vi "Fetch&Process_Measurements_V4.vi"(0 "DCPowerInformation_byChannel":T1(array[cluster]), 5 "Initial Time":timestamp, 11 "error in (no error)":errorcluster) -> (3 "Latest Time":timestamp, 4 "Data As dbl Array":dbl[][][](array[numeric]), 6 "Channel Number Array":string[](array[string]), 8 "Current Waveform Array":waveform(dbl)[](array[waveform]), 10 "Voltage Waveform Array":waveform(dbl)[](array[waveform]), 14 "TimeStamp Array":timestamp[](array[timestamp]), 15 "error out":errorcluster)   [LabVIEW 2019]
uses:
  <vilib>/Analysis/1siggen.llb/Ramp Pattern by Delta.vi
  <vilib>/Analysis/NI_AALBase.lvlib
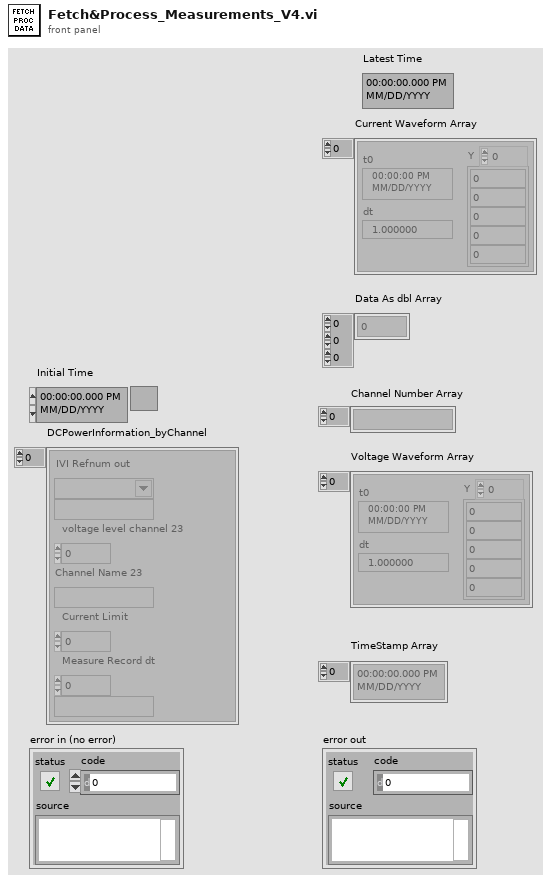
[diagram p1: front panel]
types:
  T1 = cluster{"IVI Refnum out":refnum<k15>, string, "voltage level channel 23":dbl, "Channel Name 23":string, "Current Limit":dbl, "Measure Record dt":dbl, string}[]
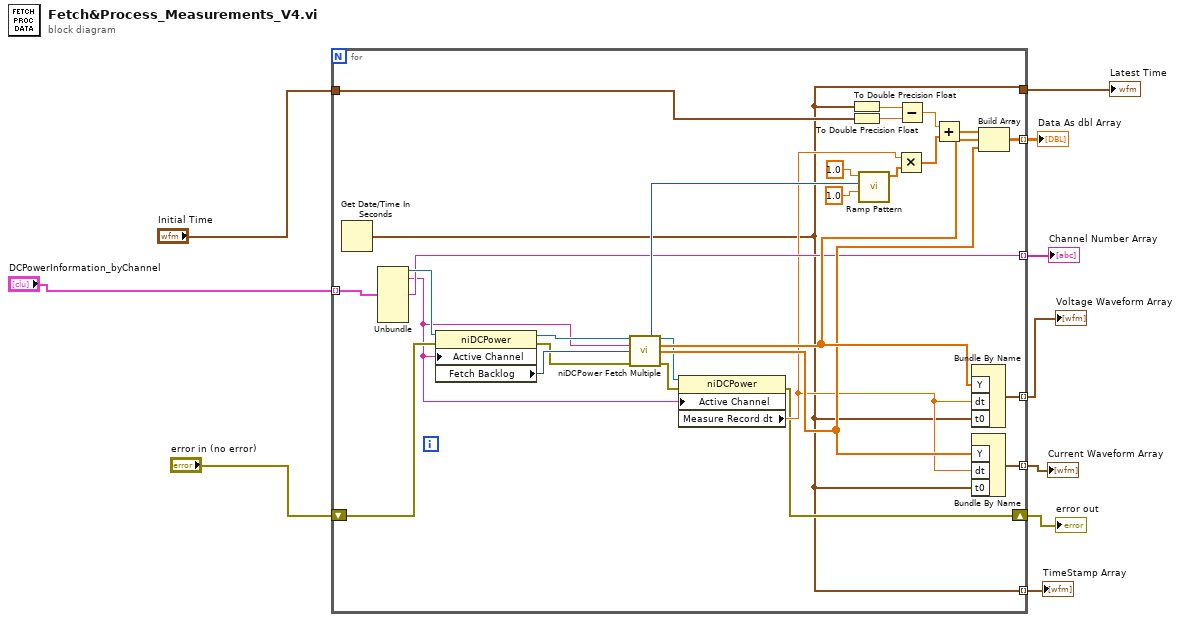
[diagram p0: block diagram]
diagram:
  n1 = for {
    tunnel: "DCPowerInformation_byChannel" -> [w15] mode=indexing
    tunnel: [w33] -> w6 mode=indexing
    tunnel: [w32] -> w7 mode=indexing
    shift-right: [w12] -> w5
    shift-left: "error in (no error)" -> [w37]
    tunnel: "Initial Time" -> [w20]
    tunnel: [w19] -> w9 mode=indexing
    tunnel: [w18] -> w10 mode=indexing
    tunnel: [w11] -> w3
    tunnel: [w11] -> w2 mode=indexing
    n2 = Get Date/Time In Seconds() -> (seconds since 1Jan1904=w11:timestamp)
    n3 = Unbundle(w15) -> ("IVI Refnum out"=w36:refnum<k15>, w13:string, "Channel Name 23"=w18:string)  [unwired: 4 out]
    n4 = property class="niDCPower"(reference=w36, error in=w37, "Active Channel"=w13) -> (reference out=w35:refnum<k15>, error out=w34:errorcluster, "Fetch Backlog"=w38:i32)
    n5 = call <instrlib>:"niDCPower Fetch Multiple.vi"("instrument handle"=w35, "channel name"=w13, "count (1)"=w38, "error in (no error)"=w34) -> ("actual count"=w21:i32, "instrument handle out"=w17:refnum<k15>, "voltage measurements"=w23:dbl[], "current measurements"=w22:dbl[], "error out"=w16:errorcluster)  [unwired: 6 in, 1 out]
    n6 = property class="niDCPower"(reference=w17, error in=w16, "Active Channel"=w13) -> (error out=w12:errorcluster, "Measure Record dt"=w14:dbl)  [unwired: 1 out]
    n7 = To Double Precision Float(number=w11) -> (double precision float=w29:dbl)
    n8 = To Double Precision Float(number=w20) -> (double precision float=w28:dbl)
    n9 = call-poly <vilib>:"Ramp Pattern.vi"("start"=1.0, "end"=w21, "delta"=1.0) -> ("Ramp Pattern"=w25:dbl[])  [unwired: 6 in, 2 out]
    n10 = Multiply(x=w14, y=w25) -> (x*y=w24:dbl[])
    n11 = Subtract(x=w29, y=w28) -> (x-y=w26:dbl)
    n12 = Add(x=w26, y=w24) -> (x+y=w31:dbl[])
    n13 = Bundle By Name("Y"=w23, "dt"=w14, "t0"=w11) -> (w33:waveform(dbl))  [unwired: 1 out]
    n14 = Bundle By Name("Y"=w22, "dt"=w14, "t0"=w11) -> (w32:waveform(dbl))  [unwired: 1 out]
    n15 = Build Array(w31, w23, w22) -> (w19:dbl[][])
  }
  "Channel Number Array" <- w10
  "Data As dbl Array" <- w9
  "Current Waveform Array" <- w7
  "Voltage Waveform Array" <- w6
  "error out" <- w5
  "Latest Time" <- w3
  "TimeStamp Array" <- w2
